vi "New Demo Filter.vi"(8 "error in (no error)":errorcluster, 11 "regular expression":string) -> (0 "error out":errorcluster, 3 "Filter Demo out":refnum<class "Filter Demo.lvclass">)   [LabVIEW 2020, in "BlueTreeMapExamples OpenSource.lvlib" / "Filter Demo.lvclass"]
uses:
  Filter Demo.lvclass
  Filter Demo.lvclass/Filter Demo.ctl
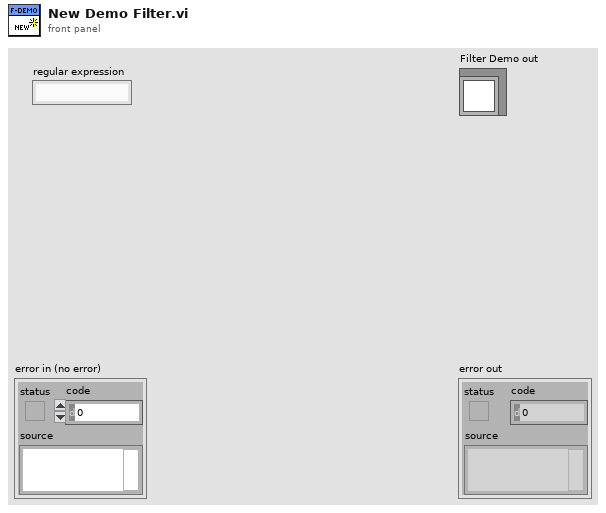
[diagram p1: front panel]
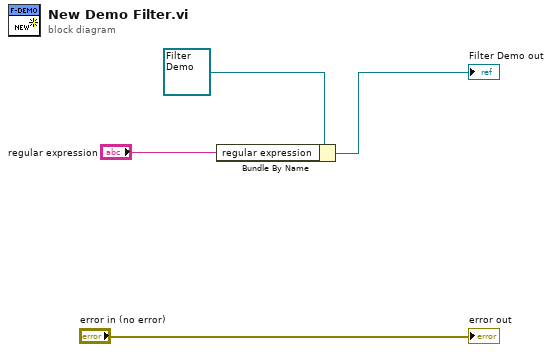
[diagram p0: block diagram]
diagram:
  n1 = Bundle By Name(cluster=refnum<class "Filter Demo.lvclass"> refnum ("Filter Demo out"), "regular expression"="regular expression") -> (→"Filter Demo out":refnum<class "Filter Demo.lvclass">)
  "error out" <- "error in (no error)"
